vi "to string array.vi"(8 "error in (no error)":errorcluster, 11 "PID Module 2 configuration in":refnum<class "PID Module 2 configuration.lvclass">) -> (0 "error out":errorcluster, 1 "Array":string[][](array[string]), 2 "version":string, 3 "PID Module 2 configuration out":refnum<class "PID Module 2 configuration.lvclass">)   [LabVIEW 2015, in "PID Module 2 configuration.lvclass"]
uses:
  PID Module 2 configuration.lvclass
  PID Module 2 configuration.lvclass/PID Module 2 configuration.ctl
  Read Lines.vi
  <vilib>/NI/Tag Bus/tag/default value polymorphs/read default value Double.vi
  <vilib>/NI/Tag Bus Module Framework/channel/TBM channel.lvclass
  <vilib>/NI/Tag Bus/tag/tag descriptor.lvclass
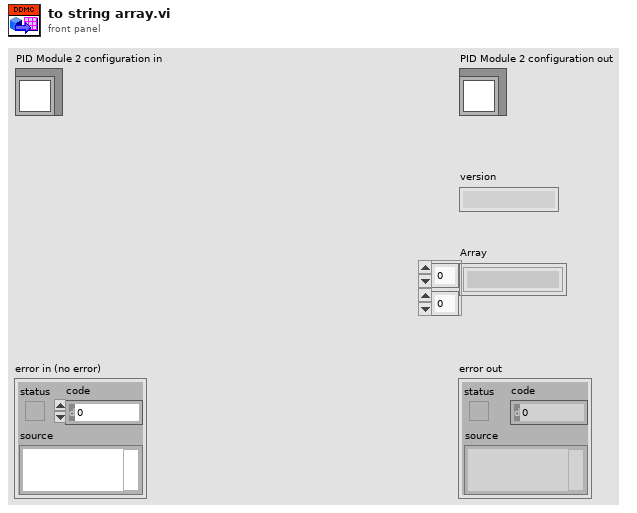
[diagram p1: front panel]
types:
  T1 = typedef "PID Module 2 configuration.lvclass/Line.ctl" = cluster{"PID ID":string, "Setpoint":refnum<class "TBM channel.lvclass">, "Variable":refnum<class "TBM channel.lvclass">, "Output":refnum<class "TBM channel.lvclass">, "Output High":refnum<class "TBM channel.lvclass">, "Output Low":refnum<class "TBM channel.lvclass">, "P":refnum<class "TBM channel.lvclass">, "I":refnum<class "TBM channel.lvclass">, "D":refnum<class "TBM channel.lvclass">}
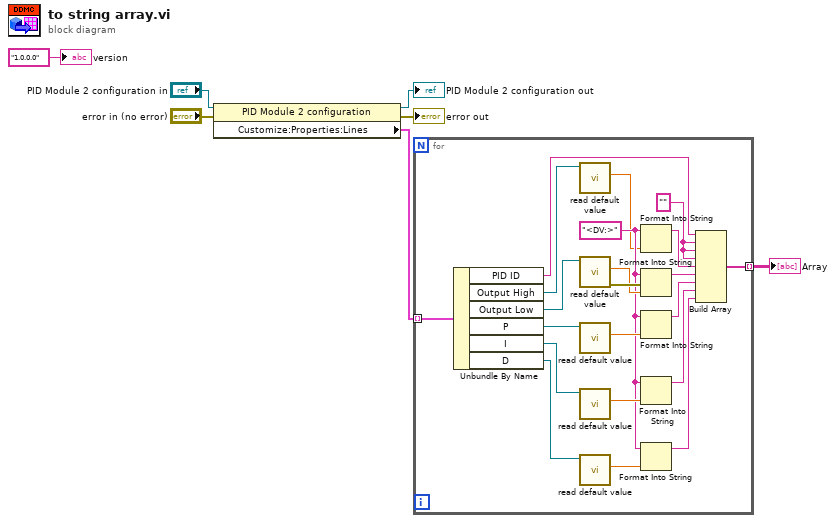
[diagram p0: block diagram]
diagram:
  n1 = property class="PID Module 2 configuration"(reference="PID Module 2 configuration in", error in="error in (no error)") -> (reference out=→"PID Module 2 configuration out":refnum<class "PID Module 2 configuration.lvclass">, error out=→"error out":errorcluster, "Customize:Properties:Lines"=w4:T1[])
  n2 = for {
    tunnel: w4 -> [w28] mode=indexing
    tunnel: [w27] -> w1 mode=indexing
    w14 = "<DV:>" ("initial string")
    w24 = "" ("element")
    n3 = Unbundle By Name(w28) -> ("PID ID"=w26:string, "Output High"=w25:refnum<class "TBM channel.lvclass">, "Output Low"=w23:refnum<class "TBM channel.lvclass">, "P"=w22:refnum<class "TBM channel.lvclass">, "I"=w21:refnum<class "TBM channel.lvclass">, "D"=w20:refnum<class "TBM channel.lvclass">)
    n4 = call-poly <vilib>:"read default value.vi"("system tag in"=w25) -> ("default value"=w8:dbl)  [unwired: 7 in, 3 out]
    n5 = call-poly <vilib>:"read default value.vi"("system tag in"=w23) -> ("error out"=w19:errorcluster, "default value"=w15:dbl)  [unwired: 7 in, 2 out]
    n6 = call-poly <vilib>:"read default value.vi"("system tag in"=w22) -> ("default value"=w16:dbl)  [unwired: 7 in, 3 out]
    n7 = call-poly <vilib>:"read default value.vi"("system tag in"=w21) -> ("default value"=w17:dbl)  [unwired: 7 in, 3 out]
    n8 = call-poly <vilib>:"read default value.vi"("system tag in"=w20) -> ("default value"=w18:dbl)  [unwired: 7 in, 3 out]
    n9 = Format Into String(initial string=w14, w8) -> (resulting string=w13:string)  [unwired: 2 in, 1 out]
    n10 = Format Into String(initial string=w14, error in=w19, w15) -> (resulting string=w12:string)  [unwired: 1 in, 1 out]
    n11 = Format Into String(initial string=w14, w16) -> (resulting string=w11:string)  [unwired: 2 in, 1 out]
    n12 = Format Into String(initial string=w14, w17) -> (resulting string=w10:string)  [unwired: 2 in, 1 out]
    n13 = Format Into String(initial string=w14, w18) -> (resulting string=w9:string)  [unwired: 2 in, 1 out]
    n14 = Build Array(w26, w24, w24, w24, w13, w12, w11, w10, w9) -> (w27:string[])
  }
  "Array" <- w1
  "version" <- "1.0.0.0" ("version")
